vi "Timing Channels RTM.vi"(8 "error in (no error)":errorcluster, 11 "Node Ptr":u64 format="%.0x") -> (0 "error out":errorcluster)   [LabVIEW 2020, in "Ballard MIL-STD-1553 System Explorer.lvlib" / "Implementation.lvlib"]
uses:
  Implementation.lvlib
  Scripting/Ballard MIL-STD-1553 Scripting.lvlib
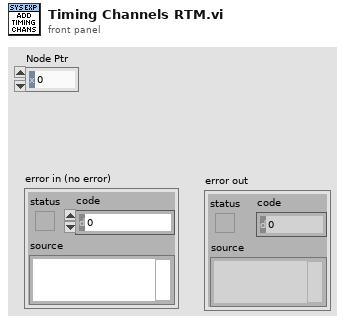
[diagram p1: front panel]
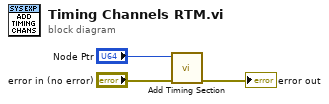
[diagram p0: block diagram]
diagram:
  n1 = call "Add Timing Section.vi"("error in"="error in (no error)", "custom device in"="Node Ptr") -> ("error out"=→"error out":errorcluster)  [unwired: 7 in, 2 out]
